vi "setParameters.vi"(0 "Game in":refnum<class "Game.lvclass">, 1 "TestMode":bool, 2 "PID gains Lateral":cluster{"(Kc)":dbl, "(Ki)":dbl, "(Kd)":dbl}, 3 "Tests":enum16{"zigzag", "goto"}(ring), 4 "PID gains Angle":cluster{"(Kc)":dbl, "(Ki)":dbl, "(Kd)":dbl}, 5 "zigzag Points":cluster{"x":dbl, "y":dbl, "Angle":dbl}[](array[cluster]), 6 "AI Parameters":T1={"Defensive Marker"=enum."SecondMostDangerous", "TimeoutDistanceInX"=0.0, "TimeoutDistanceInY"=0.0, "DistanceForaStillBall"=0.0, "TouchDistance"=0.0, "AttackerFarback"=0.0, "MinDistToKick"=0.0, "Type of Marker"=enum."BlockEnemyPass", "Type of Defense "=enum."Barreira", "PassAngle"=0.0, "KickRange"=0.0, "KickForce"=0.0, "KickEps"=0.0, "KickAngle"=0.0, "Force++"=0.0, "DistanceToKickingAngle"=0.0, "DistanceToBallOut"=0.0, "DistanceStop"=0.0, "DistanceBehindAttacker"=0.0, "Area"=enum."Circular", "DistanceForPossession"=0.0, "DistanceToConsirerRobotArrive"=0.0, "DistanceToGoAroundBall"=0.0, "DistanceInFrontOfAttacker"=0.0, "TimeoutDistanceBetweenRobots"=0.0, "MaxOutputAngle"=0.0, "MaxOutputXY"=0.0, "MaxDeceleration"=0.0, "MaxControlIncrement"=0.0, "MaxAcceleration"=0.0, "AngularToleranceForPossession"=0.0, "MaxVelBallToBeginDuelist"=0.0, "ZigZagAngle"=0.0, "PID gains Vel"={"(Kc)"=0.0, "(Ti, min)"=0.0, "(Td, min)"=0.0}, "Number of Offensive"=enum."6", "Shoot Out?"=FALSE, "DefenseAvoidArea"=FALSE, "InvertKick"=[], "Simple Pass"=FALSE, "ShootOutForce"=0.0, "dtPosEstBall"=0.0, "AttkIgnoreBallObst"=0.0, "BarrierDist"=0.0, "PassReceiver"=enum."Auto", "GoalieInFrontGoal"=0.0, "RollToPass"=FALSE, "PassReceiver"=enum."Striker", "OldRRT"=FALSE, "Dribbler"=FALSE, "VelNearBall"=0.0, "ChipKick Force"=0.0, "ForcePass\nInGame"=0.0, "bangBangParameters"={"MaxVSent"=0.0, "MaxVNorm"=0.0, "MaxVAng"=0.0, "VAngCircle"=0.0, "LBeginCircle"=0.0, "DistToDestOrientation"=0.0, "MaxVAngToTurn"=5.0, "AtkDistToDestOrientation"=4000.0}, "BallVelToAbortPass"=0.0, "BallVelToFinishPass"=0.0, "minDistanceToPass"=0.0, "dribbler_rpm"=0.0, "AttackerAngle\nToTurnInDegrees"=0.0, "AttackerAngle\nToShootInDegrees"=0.0, "distToActivateDibbler"=0.0, "StopVelocity"=3.5, "timeoutToShoot"=0.0}, 7 "PID gains Angle To Turn":cluster{"(Kc)":dbl, "(Ki)":dbl, "(Kd)":dbl}={"(Kc)"=0.0, "(Ki)"=0.3, "(Kd)"=1.0}, 8 "Project":T5, 9 "AttakingOurselves":bool, 10 "Defensive ids":dbl[](array[numeric]), 11 "ChipKick activated":bool, 12 "TestMode IDS":dbl[](array[numeric]), 13 "Debug":bool, 14 "Offensive ids":dbl[](array[numeric]), 15 "PID gains Vel D":cluster{"(Kp)":dbl, "(Ki)":dbl, "(Kd)":dbl}, 16 "Test":bool) -> (20 "Game out":refnum<class "Game.lvclass">, 27 "error out":errorcluster)   [LabVIEW 2020, in "Game.lvclass"]
uses:
  Game.lvclass
  Parameters_class/Project.ctl
  Controls/PhoenixParameters.ctl
  Play_class/PassReceiver.ctl
  Parameters_class/ChoosePassReceiver.ctl
  Navigation/Controls/bangBangControlParameters.ctl
  Game.lvclass/Game.ctl
  Parameters_class/Parameters.lvclass/Parameters.ctl
  Write Offensive ids.vi
  Write Defensive ids.vi
  Read Parameters.lvclass.vi
  Write TestMode IDs.vi
  Write TestMode.vi
  Write Tests.vi
  Parameters_class/Write Area.vi
  Parameters_class/Write DistanceBehindAttacker.vi
  Parameters_class/Write DistanceInFrontOfAttacker.vi
  Parameters_class/Write DistanceStop.vi
  Parameters_class/Write DistanceToBallOut.vi
  Parameters_class/Write DistanceToGoAroundBall.vi
  Parameters_class/Write DistanceToConsiderRobotArrive.vi
  Parameters_class/Write DistanceToKickingAngle.vi
  Parameters_class/Write Force++.vi
  Parameters_class/Write KickAngle.vi
  Parameters_class/Write KickEps.vi
  Parameters_class/Write KickForce.vi
  Parameters_class/Write KickRange.vi
  Parameters_class/Write MaxAcceleration.vi
  Parameters_class/Write MaxControlIncrement.vi
  Parameters_class/Write MaxDeceleration.vi
  Parameters_class/Write MaxOutputAngle.vi
  Parameters_class/Write MaxOutputXY.vi
  Parameters_class/Write MinDistToKick.vi
  Parameters_class/Write PassAngle.vi
  Parameters_class/Write Type of Marker.vi
  Parameters_class/Write AttackerFarback.vi
  Parameters_class/Write TouchDistance.vi
  Parameters_class/Write TimeoutDistanceInY.vi
  Parameters_class/Write TimeoutDistanceInX.vi
  Parameters_class/Write TimeoutDistanceBetweenRobots.vi
  Parameters_class/Write DistanceForPossession.vi
  Parameters_class/Write DistanceForaStillBall.vi
  Parameters_class/Write AngularToleranceForPossession.vi
  Parameters_class/Write AttakingOurselves.vi
  Parameters_class/Write Debug.vi
  Parameters_class/Write ChipKick activated.vi
  Parameters_class/Write Angle.vi
  Parameters_class/Write PID gains Vel.vi
  Parameters_class/Write PID gains Vel_desired.vi
  Parameters_class/Write PID gains Angle.vi
  Parameters_class/Write PID gains Angle To Turn.vi
  Parameters_class/Write Number of Offesnive.vi
  Parameters_class/Write Shoot Out_.vi
  Parameters_class/Write DefenseAvoidArea.vi
  Parameters_class/Write InvertKick.vi
  Parameters_class/Write SimplePass.vi
  Parameters_class/Write ShootOutForce.vi
  Parameters_class/Write dtPosEstBall.vi
  Parameters_class/Write PassReceiver.vi
  Parameters_class/Write GoalieInFrontGoal.vi
  Parameters_class/Write RollToPass.vi
  Parameters_class/Write Project.vi
  Parameters_class/Write Dribbler.vi
  Parameters_class/Write VelNearBall.vi
  Parameters_class/Write ChipKick Force.vi
  Parameters_class/Write ForceInGame.vi
  Parameters_class/Write bangBangParameters.vi
  Parameters_class/Write BallVelToAbortPass.vi
  Parameters_class/Write BallVelToFinishPass.vi
  Parameters_class/Write minDistanceToPass.vi
  Parameters_class/Write dribbler_rpm.vi
  Parameters_class/Write StopVelocity.vi
  Parameters_class/Write timeoutToShoot.vi
  Write Parameters.lvclass.vi
  Parameters_class/Write AttackerAngleToTurnInDegrees.vi
  Parameters_class/Write AttackerAngleToShootInDegrees.vi
  Parameters_class/Parameters.lvclass
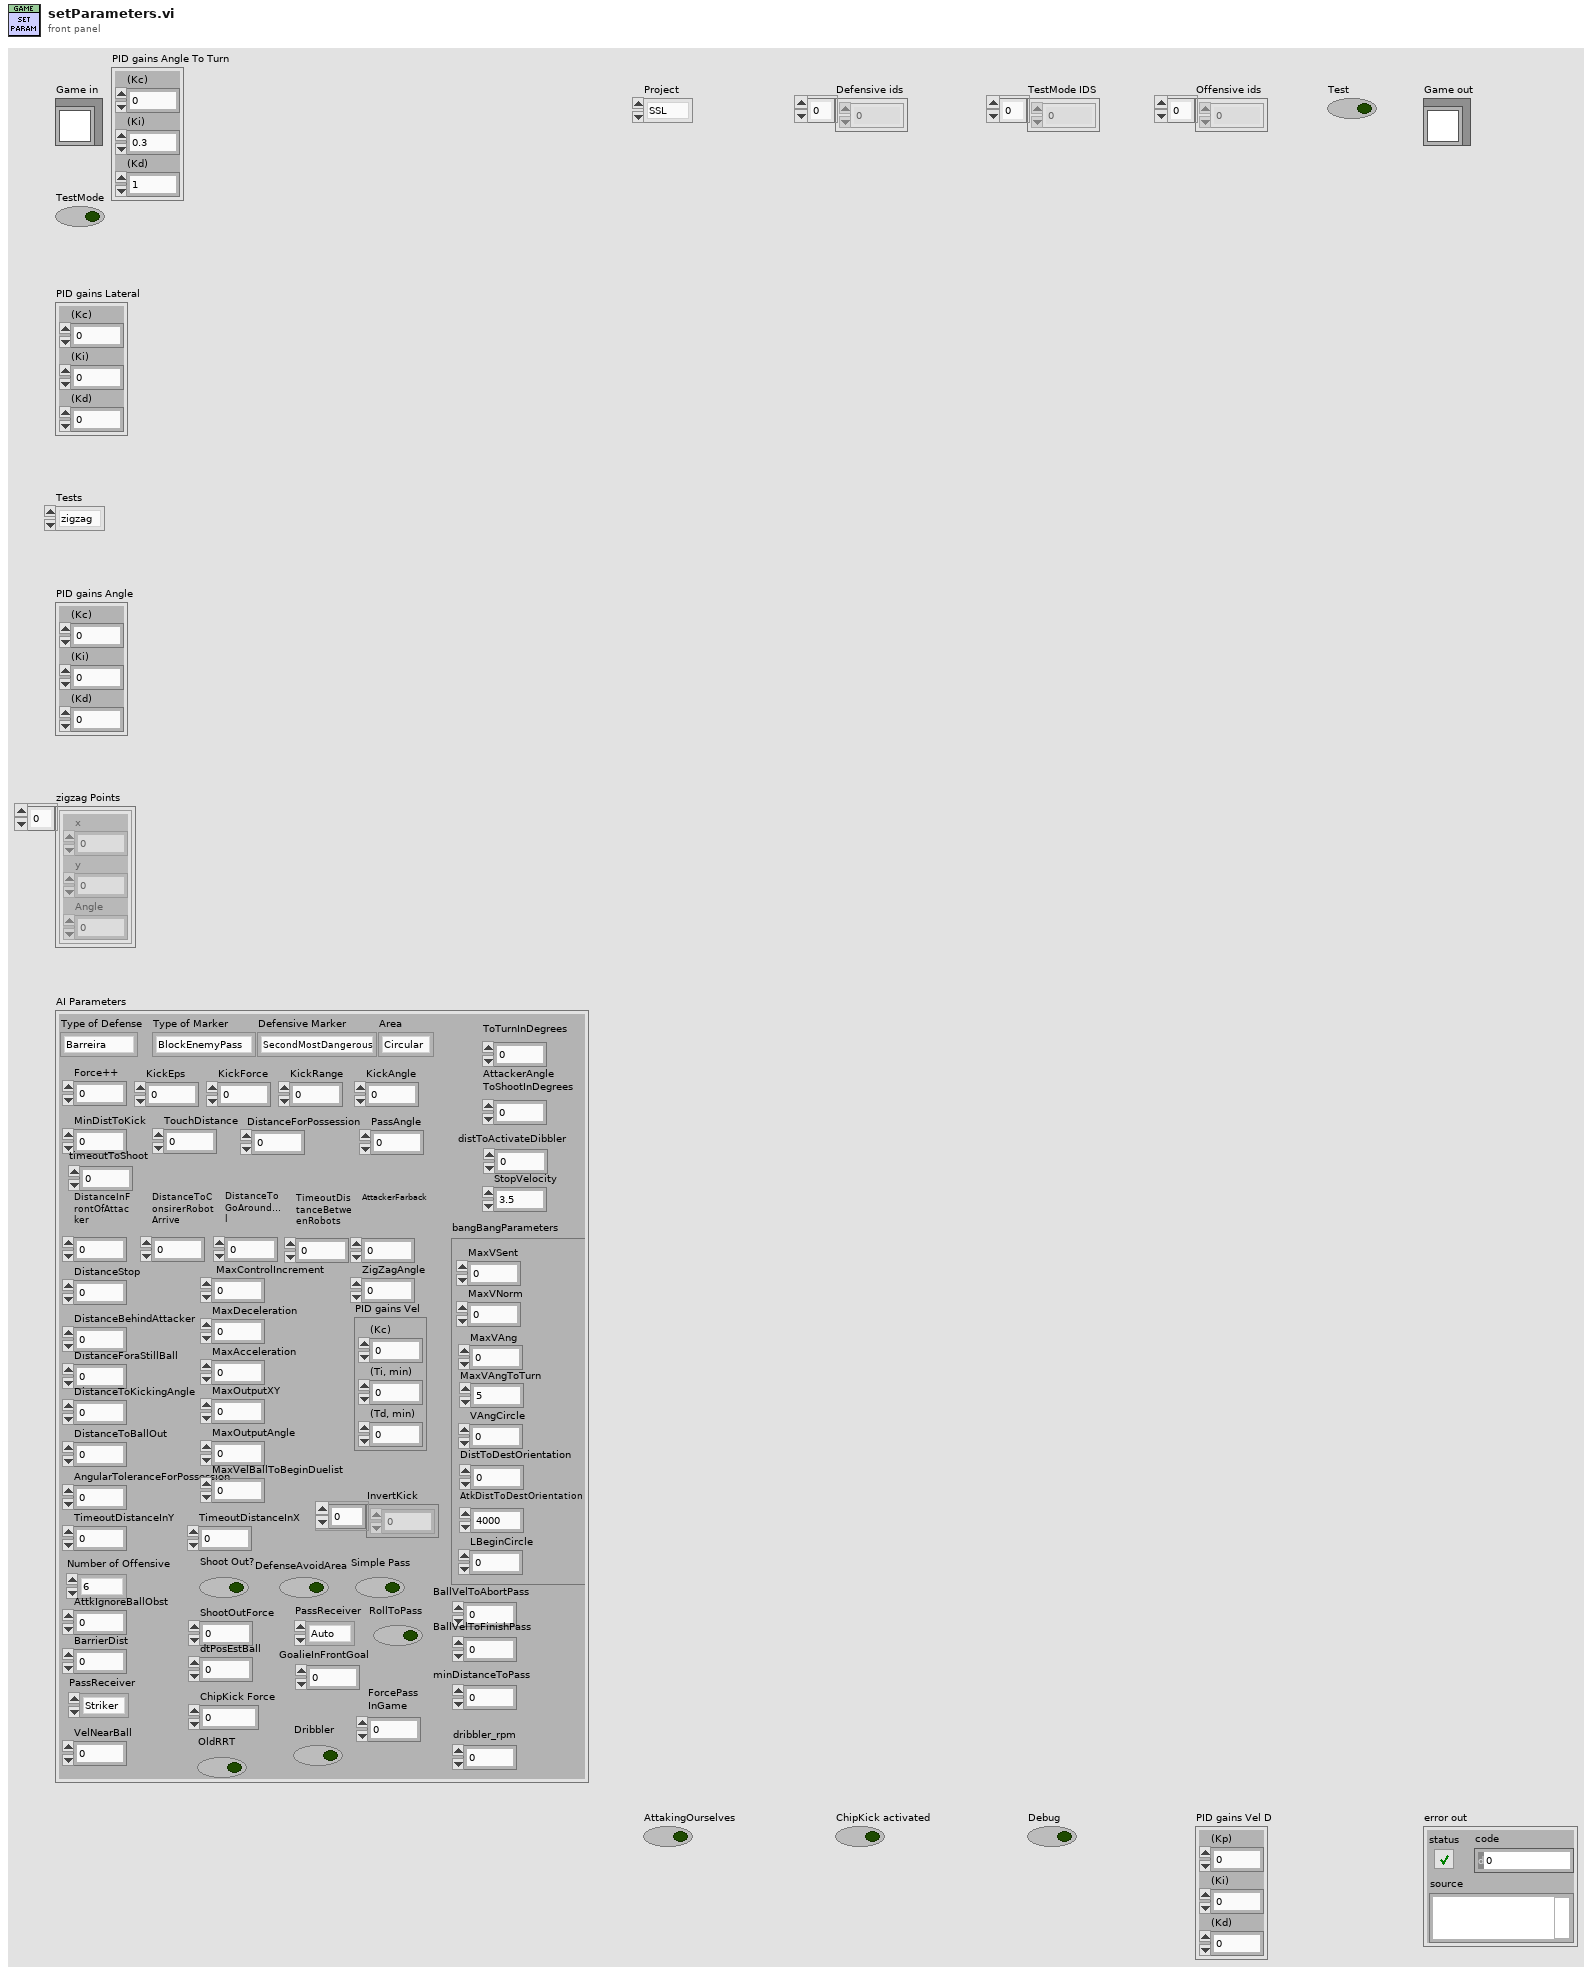
[diagram p1: front panel]
types:
  T1 = typedef "PhoenixParameters.ctl" = cluster{"Defensive Marker":enum16{"SecondMostDangerous", "MostDangerous"}, "TimeoutDistanceInX":dbl, "TimeoutDistanceInY":dbl, "DistanceForaStillBall":dbl, "TouchDistance":dbl, "AttackerFarback":dbl, "MinDistToKick":dbl, "Type of Marker":enum16{"BlockEnemyPass", "BlockOurGoal"}, "Type of Defense ":enum16{"Barreira", "Manmark"}, "PassAngle":dbl, "KickRange":dbl, "KickForce":dbl, "KickEps":dbl, "KickAngle":dbl, "Force++":dbl, "DistanceToKickingAngle":dbl, "DistanceToBallOut":dbl, "DistanceStop":dbl, "DistanceBehindAttacker":dbl, "Area":enum16{"Circular", "Square"}, "DistanceForPossession":dbl, "DistanceToConsirerRobotArrive":dbl, "DistanceToGoAroundBall":dbl, "DistanceInFrontOfAttacker":dbl, "TimeoutDistanceBetweenRobots":dbl, "MaxOutputAngle":dbl, "MaxOutputXY":dbl, "MaxDeceleration":dbl, "MaxControlIncrement":dbl, "MaxAcceleration":dbl, "AngularToleranceForPossession":dbl, "MaxVelBallToBeginDuelist":dbl, "ZigZagAngle":dbl, "PID gains Vel":cluster{"(Kc)":dbl, "(Ti, min)":dbl, "(Td, min)":dbl}, "Number of Offensive":enum16{"6", "5", "4", "3", "2", "1", "0", "Auto"}, "Shoot Out?":bool, "DefenseAvoidArea":bool, "InvertKick":dbl[], "Simple Pass":bool, "ShootOutForce":dbl, "dtPosEstBall":dbl, "AttkIgnoreBallObst":dbl, "BarrierDist":dbl, "PassReceiver":T2, "GoalieInFrontGoal":dbl, "RollToPass":bool, "PassReceiver":T3, "OldRRT":bool, "Dribbler":bool, "VelNearBall":dbl, "ChipKick Force":dbl, "ForcePass\nInGame":dbl, "bangBangParameters":T4, "BallVelToAbortPass":dbl, "BallVelToFinishPass":dbl, "minDistanceToPass":dbl, "dribbler_rpm":dbl, "AttackerAngle\nToTurnInDegrees":dbl, "AttackerAngle\nToShootInDegrees":dbl, "distToActivateDibbler":dbl, "StopVelocity":dbl, "timeoutToShoot":dbl}
  T2 = typedef "PassReceiver.ctl" = enum16{"Auto", "2ndStriker", "Striker"}
  T3 = typedef "ChoosePassReceiver.ctl" = enum16{"Striker", "2ndStriker", "Auto"}
  T4 = typedef "bangBangControlParameters.ctl" = cluster{"MaxVSent":dbl, "MaxVNorm":dbl, "MaxVAng":dbl, "VAngCircle":dbl, "LBeginCircle":dbl, "DistToDestOrientation":dbl, "MaxVAngToTurn":dbl, "AtkDistToDestOrientation":dbl}
  T5 = typedef "Project.ctl" = enum16{"SSL", "VSS"}
  T6 = cluster{"(Kc)":dbl, "(Ti, min)":dbl, "(Td, min)":dbl}
  T7 = enum16{"6", "5", "4", "3", "2", "1", "0", "Auto"}
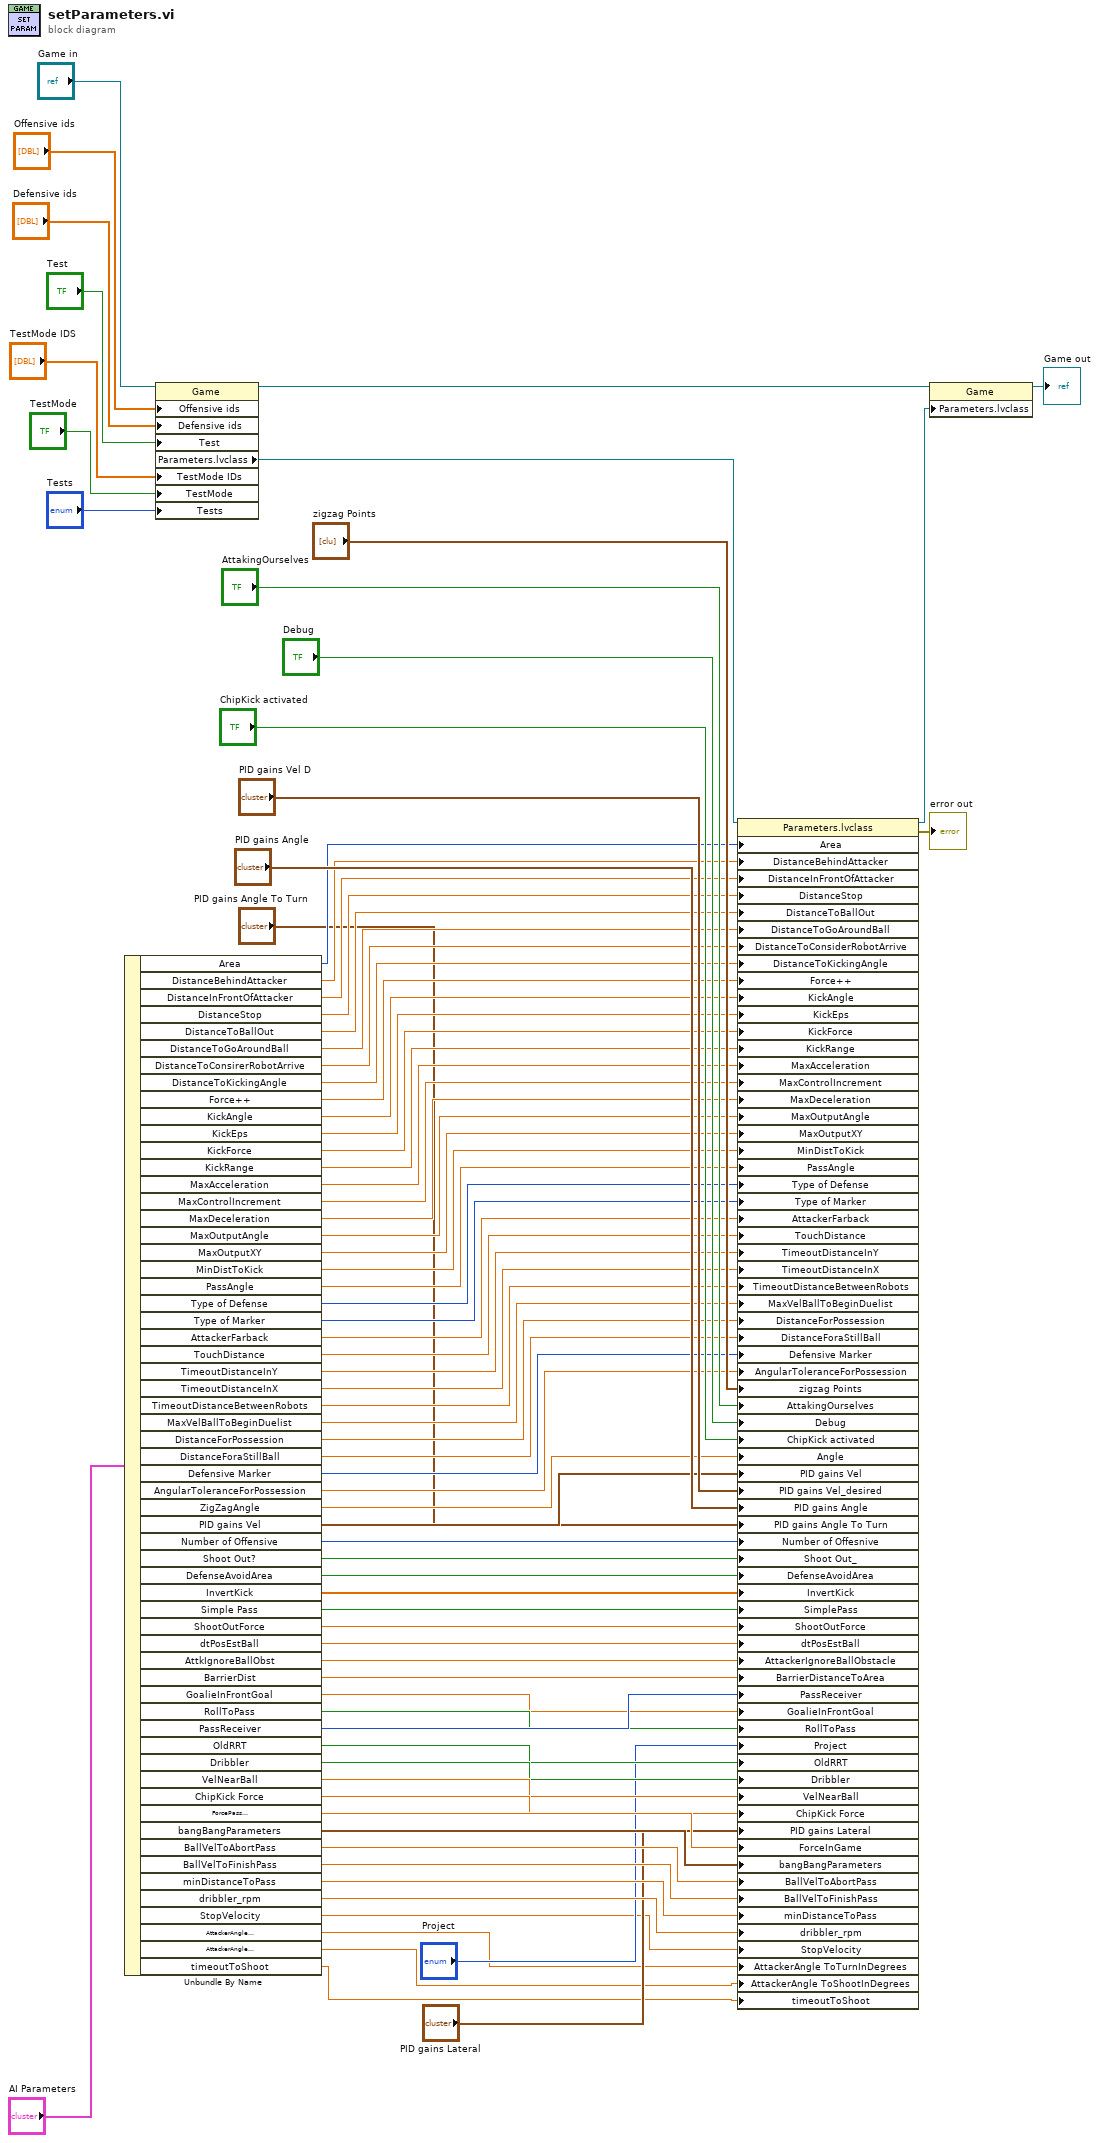
[diagram p0: block diagram]
diagram:
  n1 = Unbundle By Name("AI Parameters") -> ("Area"=w19:enum16{"Circular", "Square"}, "DistanceBehindAttacker"=w20:dbl, "DistanceInFrontOfAttacker"=w21:dbl, "DistanceStop"=w22:dbl, "DistanceToBallOut"=w23:dbl, "DistanceToGoAroundBall"=w24:dbl, "DistanceToConsirerRobotArrive"=w25:dbl, "DistanceToKickingAngle"=w50:dbl, "Force++"=w49:dbl, "KickAngle"=w48:dbl, "KickEps"=w47:dbl, "KickForce"=w46:dbl, "KickRange"=w45:dbl, "MaxAcceleration"=w44:dbl, "MaxControlIncrement"=w43:dbl, "MaxDeceleration"=w42:dbl, "MaxOutputAngle"=w41:dbl, "MaxOutputXY"=w40:dbl, "MinDistToKick"=w39:dbl, "PassAngle"=w38:dbl, "Type of Defense"=w37:enum16{"Barreira", "Manmark"}, "Type of Marker"=w36:enum16{"BlockEnemyPass", "BlockOurGoal"}, "AttackerFarback"=w35:dbl, "TouchDistance"=w34:dbl, "TimeoutDistanceInY"=w33:dbl, "TimeoutDistanceInX"=w32:dbl, "TimeoutDistanceBetweenRobots"=w31:dbl, "MaxVelBallToBeginDuelist"=w30:dbl, "DistanceForPossession"=w29:dbl, "DistanceForaStillBall"=w28:dbl, "Defensive Marker"=w27:enum16{"SecondMostDangerous", "MostDangerous"}, "AngularToleranceForPossession"=w26:dbl, "ZigZagAngle"=w53:dbl, "PID gains Vel"=w55:T6, "Number of Offensive"=w58:T7, "Shoot Out?"=w60:bool, "DefenseAvoidArea"=w61:bool, "InvertKick"=w62:dbl[], "Simple Pass"=w63:bool, "ShootOutForce"=w64:dbl, "dtPosEstBall"=w65:dbl, "AttkIgnoreBallObst"=w66:dbl, "BarrierDist"=w67:dbl, "GoalieInFrontGoal"=w68:dbl, "RollToPass"=w69:bool, "PassReceiver"=w70:T3, "OldRRT"=w72:bool, "Dribbler"=w73:bool, "VelNearBall"=w74:dbl, "ChipKick Force"=w75:dbl, "ForcePass\nInGame"=w77:dbl, "bangBangParameters"=w78:T4, "BallVelToAbortPass"=w79:dbl, "BallVelToFinishPass"=w80:dbl, "minDistanceToPass"=w81:dbl, "dribbler_rpm"=w82:dbl, "StopVelocity"=w5:dbl, "AttackerAngle\nToTurnInDegrees"=w3:dbl, "AttackerAngle\nToShootInDegrees"=w2:dbl, "timeoutToShoot"=w1:dbl)
  n2 = property class="Game"(reference="Game in", "Offensive ids"="Offensive ids", "Defensive ids"="Defensive ids", "Test"="Test", "TestMode IDs"="TestMode IDS", "TestMode"="TestMode", "Tests"="Tests") -> (reference out=w10:refnum<class "Game.lvclass">, "Parameters.lvclass"=w9:refnum<class "Parameters.lvclass">)  [unwired: 1 in, 1 out]
  n3 = property class="Parameters.lvclass"(reference=w9, "Area"=w19, "DistanceBehindAttacker"=w20, "DistanceInFrontOfAttacker"=w21, "DistanceStop"=w22, "DistanceToBallOut"=w23, "DistanceToGoAroundBall"=w24, "DistanceToConsiderRobotArrive"=w25, "DistanceToKickingAngle"=w50, "Force++"=w49, "KickAngle"=w48, "KickEps"=w47, "KickForce"=w46, "KickRange"=w45, "MaxAcceleration"=w44, "MaxControlIncrement"=w43, "MaxDeceleration"=w42, "MaxOutputAngle"=w41, "MaxOutputXY"=w40, "MinDistToKick"=w39, "PassAngle"=w38, "Type of Defense"=w37, "Type of Marker"=w36, "AttackerFarback"=w35, "TouchDistance"=w34, "TimeoutDistanceInY"=w33, "TimeoutDistanceInX"=w32, "TimeoutDistanceBetweenRobots"=w31, "MaxVelBallToBeginDuelist"=w30, "DistanceForPossession"=w29, "DistanceForaStillBall"=w28, "Defensive Marker"=w27, "AngularToleranceForPossession"=w26, "zigzag Points"="zigzag Points", "AttakingOurselves"="AttakingOurselves", "Debug"="Debug", "ChipKick activated"="ChipKick activated", "Angle"=w53, "PID gains Vel"=w55, "PID gains Vel_desired"="PID gains Vel D", "PID gains Angle"="PID gains Angle", "PID gains Angle To Turn"="PID gains Angle To Turn", "Number of Offesnive"=w58, "Shoot Out_"=w60, "DefenseAvoidArea"=w61, "InvertKick"=w62, "SimplePass"=w63, "ShootOutForce"=w64, "dtPosEstBall"=w65, "AttackerIgnoreBallObstacle"=w66, "BarrierDistanceToArea"=w67, "PassReceiver"=w70, "GoalieInFrontGoal"=w68, "RollToPass"=w69, "Project"="Project", "OldRRT"=w72, "Dribbler"=w73, "VelNearBall"=w74, "ChipKick Force"=w75, "PID gains Lateral"="PID gains Lateral", "ForceInGame"=w77, "bangBangParameters"=w78, "BallVelToAbortPass"=w79, "BallVelToFinishPass"=w80, "minDistanceToPass"=w81, "dribbler_rpm"=w82, "StopVelocity"=w5, "AttackerAngle ToTurnInDegrees"=w3, "AttackerAngle ToShootInDegrees"=w2, "timeoutToShoot"=w1) -> (reference out=w12:refnum<class "Parameters.lvclass">, error out=→"error out":errorcluster)  [unwired: 1 in]
  n4 = property class="Game"(reference=w10, "Parameters.lvclass"=w12) -> (reference out=→"Game out":refnum<class "Game.lvclass">)  [unwired: 1 in, 1 out]
